vi "Add Channels Dialog.vi"() -> (2 "Update?":bool, 3 "Channel Config":T1)   [LabVIEW 2019, in "Software Multi-Plex System Explorer.lvlib"]
uses:
  Software Multi-Plex System Explorer.lvlib
  Types/Index Type.ctl
  Types/Channel Config.ctl
panel:
  in  "Cancel":bool
  in  "Add":bool
  in  "Channel Indexing":T2
  in  "Channel Prefix":string="Channel "
  in  "Inputs Per Channel":i32=3 min=2 step=1
  in  "Channels":i32=1 min=1 step=1
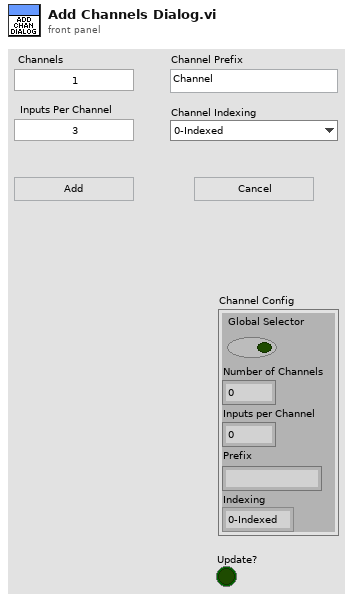
[diagram p1: front panel]
types:
  T1 = typedef "Software Multi-Plex System Explorer.lvlib/Channel Config.ctl" = cluster{"Global Selector":bool, "Number of Channels":i32, "Inputs per Channel":i32, "Prefix":string, "Indexing":T2}
  T2 = typedef "Software Multi-Plex System Explorer.lvlib/Index Type.ctl" = enum16{"0-Indexed", "1-Indexed"}
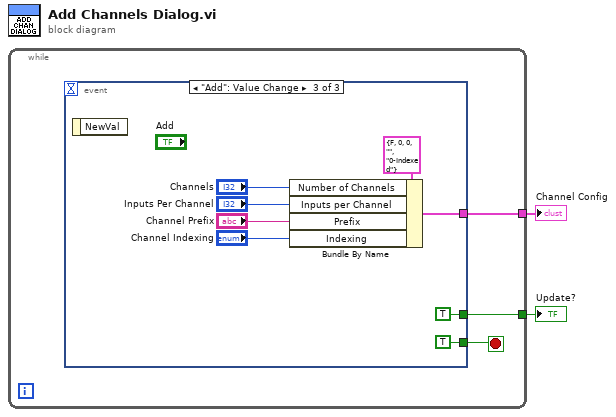
[diagram p0: block diagram]
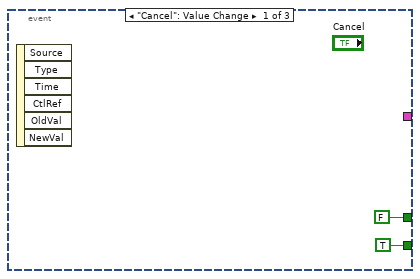
[diagram p2: hidden frame]
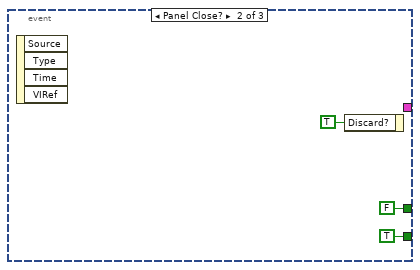
[diagram p3: hidden frame]
diagram:
  n1 = while {
    tunnel: [w4] -> w2
    tunnel: [w3] -> w1
    stop <- w5 stop-if-true
    n2 = event shown="[2] \"Add\": Value Change" {
      selector: _ -> [_ _ _]
      dyn-events: _ -> [_ _ _]
      timeout: _ -> [_ _ _]
      tunnel: [TRUE TRUE TRUE] -> w5
      tunnel: [FALSE FALSE TRUE] -> w4
      tunnel: [_ _ w11] -> w3
      event "Cancel": Value Change {
        n3 = event-data() -> ()  [unwired: 1 in, 6 out]
      }
      event Panel Close? {
        n4 = event-data() -> ()  [unwired: 1 in, 4 out]
        n5 = event-data("Discard?"=TRUE) -> ()  [unwired: 1 in, 1 out]
      }
      event "Add": Value Change {
        n6 = event-data() -> ()  [unwired: 1 in, 1 out]
        n7 = Bundle By Name(cluster=T1 {"Global Selector"=FALSE, "Number of Channels"=0, "Inputs per Channel"=0, "Prefix"="", "Indexing"=enum."0-Indexed"} ("Channel Config"), "Number of Channels"="Channels", "Inputs per Channel"="Inputs Per Channel", "Prefix"="Channel Prefix", "Indexing"="Channel Indexing") -> (w11:T1)
      }
    }
  }
  "Update?" <- w2
  "Channel Config" <- w1
